vi "(SubVI)I2C_16Bit-16Bit_Read_Sequential.vi"(5 "Log Ref":refnum<vi>, 7 "Clock":T1=enum."400kHz", 8 "error in (no error)":errorcluster caption="에러 입력(에러 없음)", 9 "Size to Read":u16, 10 "Start Address":u16, 11 "ID":u8) -> (0 "error out":errorcluster caption="에러 출력", 2 "Log":string, 3 "Read Data":u16[](array[numeric]))   [LabVIEW 2020]
uses:
  Controls/(Ctrl)I2C_Clock.ctl
  Controls/(Ctrl)I2C_RW.ctl
  Controls/(Ctrl)I2C_Data Size.ctl
  Serial/Controls/(Ctrl)Serial_Write Read Option.ctl
  Variables/(Var)System Variables.vi
  Serial/Instance VIs/(SubVI)Serial_Write-Read.vi
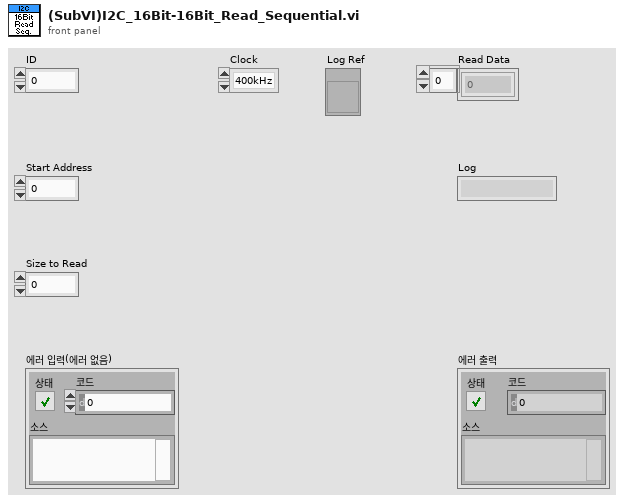
[diagram p1: front panel]
types:
  T1 = typedef "(Ctrl)I2C_Clock.ctl" = enum8{"1MHz", "2MHz", "3MHz", "400kHz"}
  T2 = typedef "(Ctrl)I2C_Data Size.ctl" = enum16{"8Bit_8Bit", "16Bit_16Bit", "16Bit_8Bit"}
  T3 = typedef "(Ctrl)I2C_RW.ctl" = enum16{"Read", "Write"}
  T4 = typedef "(Ctrl)Serial_Write Read Option.ctl" = cluster{"Echo Request":bool, "Header Verification":bool, "Checksum Verification":bool, "User Code Verifiaction":bool}
  T5 = typedef "IC I2C Clock Rate.ctl" = enum8{"50khz", "100khz", "400khz", "1Mhz", "1.2Mhz"}
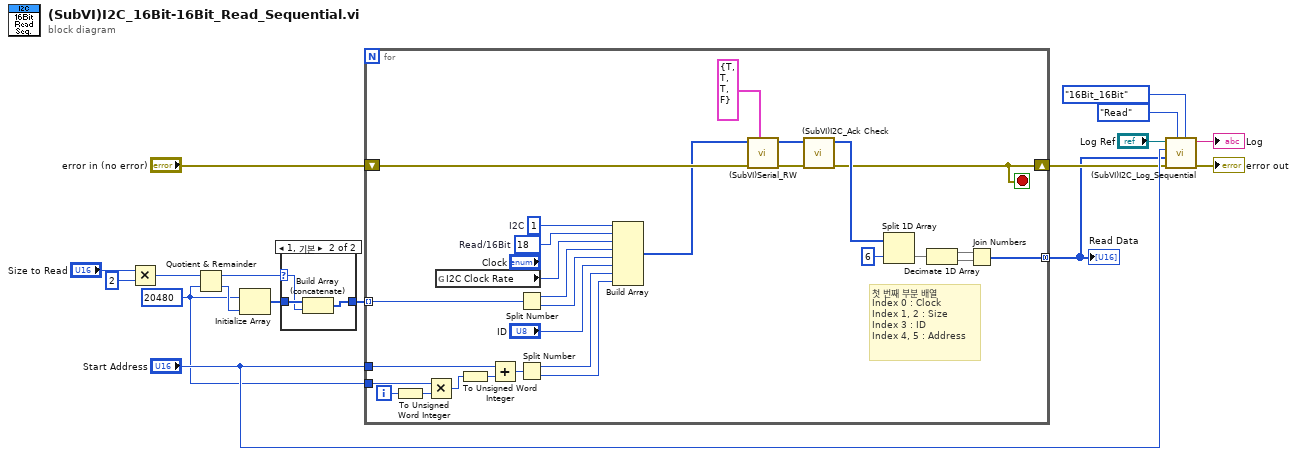
[diagram p0: block diagram]
diagram:
  w4 = u16 20480 ("y")
  n1 = Multiply(x="Size to Read", y=u16 2) -> (x*y=w2:u16)
  n2 = Quotient & Remainder(x=w2, y=w4) -> (x-y*floor(x/y)=w7:u16, floor(x/y)=w9:u16)
  n3 = Initialize Array(w4, w9) -> (w8:u16[])
  n4 = case shown="1, 기본" w7 {
    selector: w7 -> [_ w19]
    tunnel: w8 -> [w18 w21]
    tunnel: [w18 w20] -> w5
    frame 0 {
    }
    frame 1, Default {
      n5 = Build Array (concatenate)(w21, w19) -> (w20:u16[])
    }
  }
  n6 = for {
    tunnel: [w35] -> w3 mode=concatenating
    tunnel: "Start Address" -> [w25]
    tunnel: w5 -> [w31] mode=indexing
    shift-right: [w23] -> w10
    shift-left: "error in (no error)" -> [w49]
    tunnel: w4 -> [w29]
    i -> [w30]
    stop <- w23 stop-if-true
    w47 = u8 18  # Read/16Bit
    w48 = u8 1  # I2C
    # "첫 번째 부분 배열\nIndex 0 : Clock\nIndex 1, 2 : Size\nIndex 3 : ID\nIndex 4, 5 : Address"
    n7 = To Unsigned Word Integer(number=w30) -> (unsigned 16bit integer=w28:u16)
    n8 = Multiply(x=w29, y=w28) -> (x*y=w27:u16)
    n9 = global read "(Var)System Variables.vi" "I2C Clock Rate"() -> (w22:T5)
    n10 = To Unsigned Word Integer(number=w27) -> (unsigned 16bit integer=w26:u16)
    n11 = Add(x=w25, y=w26) -> (x+y=w24:u16)
    n12 = Split Number(x=w31) -> (hi(x)=w46:u8, lo(x)=w45:u8)
    n13 = Split Number(x=w24) -> (hi(x)=w40:u8, lo(x)=w41:u8)
    n14 = Build Array(w48, w47, w22, w46, w45, "ID", w40, w41) -> (w32:u8[])
    n15 = call-poly "(SubVI)Serial_RW.vi"("Option"=T4 {"Echo Request"=TRUE, "Header Verification"=TRUE, "Checksum Verification"=TRUE, "User Code Verifiaction"=FALSE}, "error in (no error)"=w49, "Data to Write"=w32) -> ("error out"=w34:errorcluster, "Read Data"=w36:u8[])  [unwired: 6 in, 1 out]
    n16 = call "(SubVI)I2C_Ack Check.vi"("에러 입력(에러 없음)"=w34, "Read Data"=w36) -> ("에러 출력"=w23:errorcluster, "Read Data Out"=w33:u8[])  [unwired: 8 in]
    n17 = Split 1D Array(array=w33, index=6 ("인덱스")) -> (second subarray=w42:u8[])  [unwired: 1 out]
    n18 = Decimate 1D Array(w42) -> (w39:u8[], w38:u8[])
    n19 = Join Numbers(hi=w39, lo=w38) -> ((hi.lo)=w35:u16[])
  }
  "Read Data" <- w3
  n20 = call "(SubVI)I2C_Log_Sequential.vi"("Data Size"=(Ctrl)I2C_Data_Size."16Bit_16Bit", "R/W"=(Ctrl)I2C_RW."Read", "error in (no error)"=w10, "Data Array"=w3, "Start Address"="Start Address", "Log Ref"="Log Ref") -> ("error out"=→"error out":errorcluster, "Log"=→"Log":string)  [unwired: 4 in]
